vi "calibinformation.vi"(0 "object in":refnum<class "MBinteractive.lvclass">, 1 "校准点信息":u16[](array[numeric]), 5 "error in (no error)":errorcluster) -> (14 "object out":refnum<class "MBinteractive.lvclass">, 19 "error out":errorcluster)   [LabVIEW 2016, in "MBinteractive.lvclass"]
uses:
  MBinteractive.lvclass
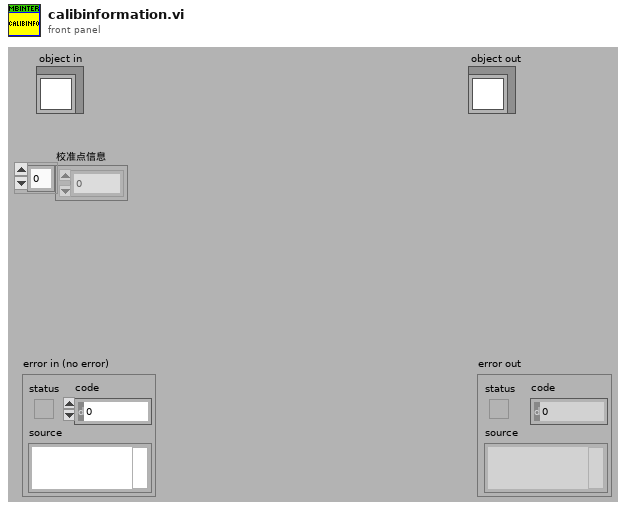
[diagram p1: front panel]
types:
  T1 = cluster{"低标液1浓度":dbl, "低标液1信号值":dbl, "低标液1启用":u16, "低标液2浓度":dbl, "低标液2信号值":dbl, "低标液2启用":u16, "低标液3浓度":dbl, "低标液3信号值":dbl, "低标液3启用":u16, "低标液4浓度":dbl, "低标液4信号值":dbl, "低标液4启用":u16, "低标液5浓度":dbl, "低标液5信号值":dbl, "低标液5启用":u16, "高标液1浓度":dbl, "高标液1信号值":dbl, "高标液1启用":u16, "高标液2浓度":dbl, "高标液2信号值":dbl, "高标液2启用":u16, "高标液3浓度":dbl, "高标液3信号值":dbl, "高标液3启用":u16, "高标液4浓度":dbl, "高标液4信号值":dbl, "高标液4启用":u16, "高标液5浓度":dbl, "高标液5信号值":dbl, "高标液5启用":u16, "低斜率":dbl, "低截距":dbl, "低二次多项式系数":dbl, "低线性相关系数":dbl, "高斜率":dbl, "高截距":dbl, "高二次多项式系数":dbl, "高线性相关系数":dbl}
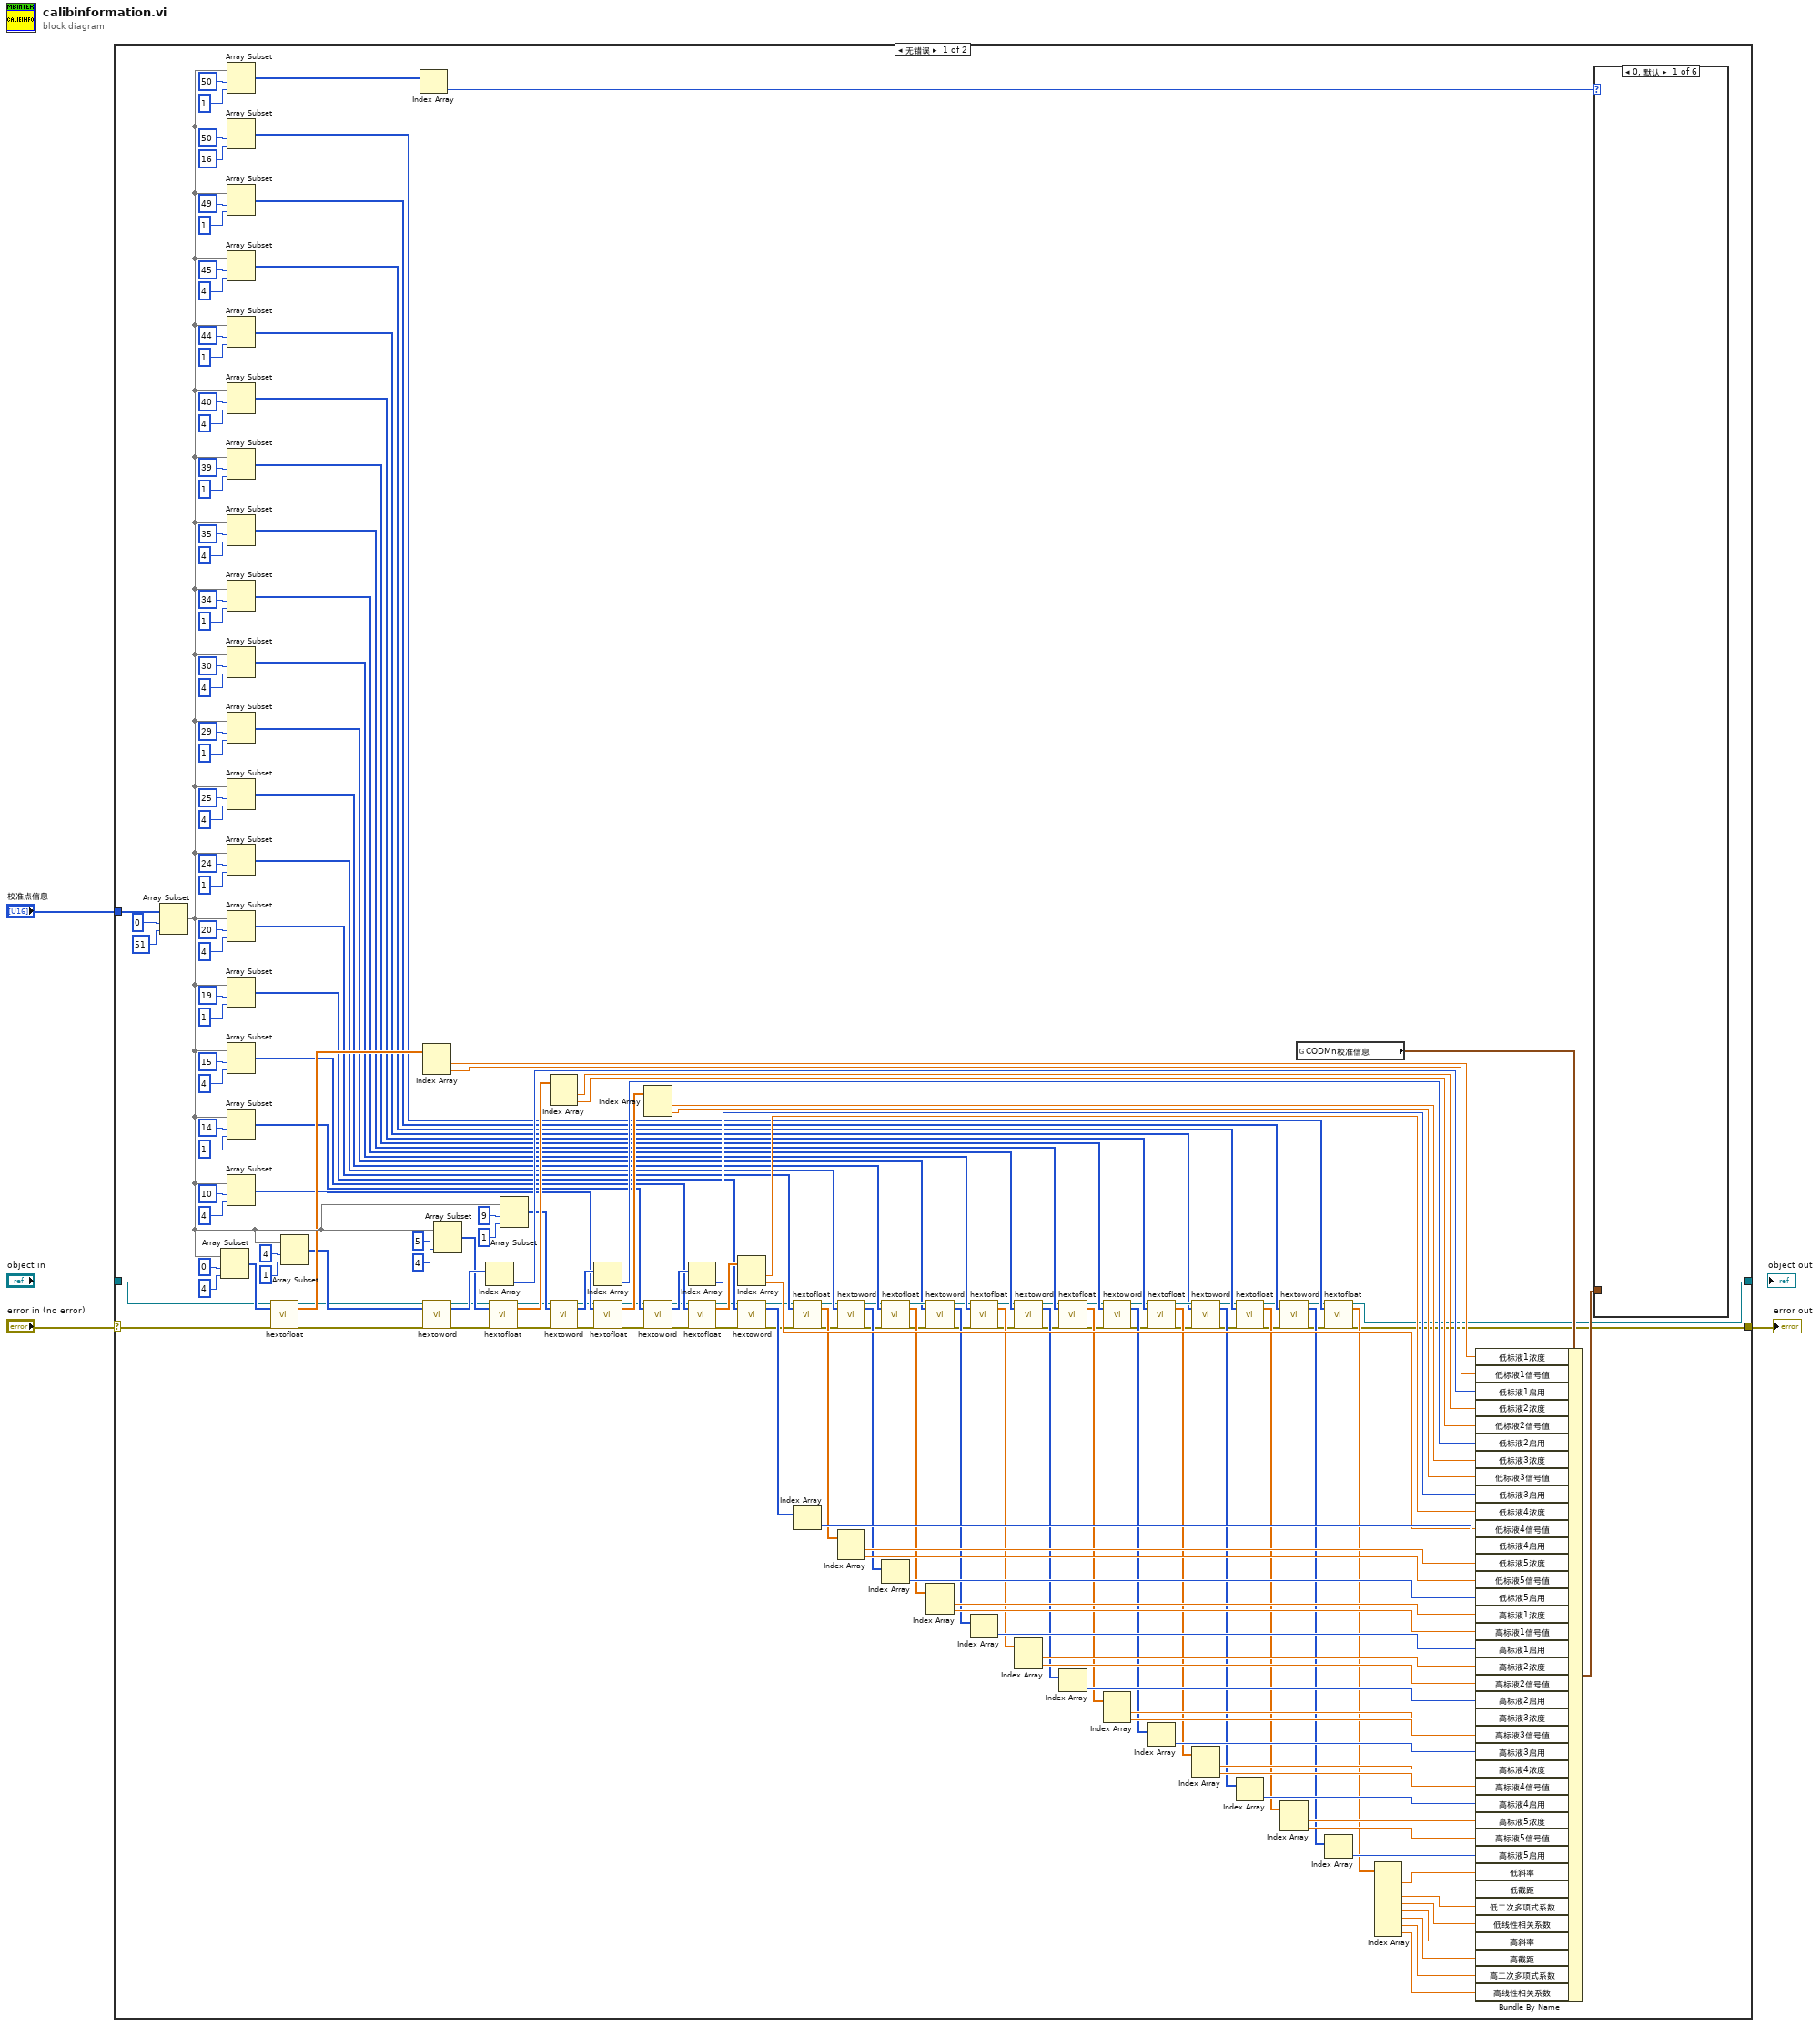
[diagram p0: block diagram]
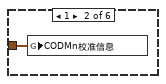
[diagram p2: hidden frame]
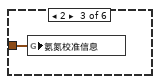
[diagram p3: hidden frame]
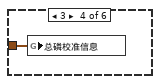
[diagram p4: hidden frame]
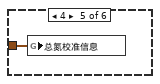
[diagram p5: hidden frame]
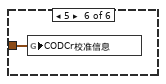
[diagram p6: hidden frame]
diagram:
  n1 = case shown="无错误" "error in (no error)" {
    selector: "error in (no error)" -> [w28 w188]
    tunnel: [w6 w188] -> w4
    tunnel: [w29 w187] -> w2
    tunnel: "object in" -> [w89 w187]
    tunnel: "校准点信息" -> [w93 _]
    frame No Error {
      n2 = Array Subset(array=w93, index=0 ("y"), length=51 ("长度")) -> (w173:u16[])
      n3 = Array Subset(array=w173, index=0 ("索引"), length=4 ("长度")) -> (w91:u16[])
      n4 = Array Subset(array=w173, index=50 ("索引"), length=1 ("长度")) -> (w170:u16[])
      n5 = Array Subset(array=w173, index=50 ("索引"), length=16 ("长度")) -> (w70:u16[])
      n6 = Array Subset(array=w173, index=49 ("索引"), length=1 ("长度")) -> (w58:u16[])
      n7 = Array Subset(array=w173, index=45 ("索引"), length=4 ("长度")) -> (w68:u16[])
      n8 = Array Subset(array=w173, index=44 ("索引"), length=1 ("长度")) -> (w34:u16[])
      n9 = Array Subset(array=w173, index=40 ("索引"), length=4 ("长度")) -> (w66:u16[])
      n10 = Array Subset(array=w173, index=39 ("索引"), length=1 ("长度")) -> (w38:u16[])
      n11 = Array Subset(array=w173, index=35 ("索引"), length=4 ("长度")) -> (w63:u16[])
      n12 = Array Subset(array=w173, index=34 ("索引"), length=1 ("长度")) -> (w42:u16[])
      n13 = Array Subset(array=w173, index=30 ("索引"), length=4 ("长度")) -> (w61:u16[])
      n14 = Array Subset(array=w173, index=29 ("索引"), length=1 ("长度")) -> (w45:u16[])
      n15 = Array Subset(array=w173, index=25 ("索引"), length=4 ("长度")) -> (w60:u16[])
      n16 = Array Subset(array=w173, index=24 ("索引"), length=1 ("长度")) -> (w56:u16[])
      n17 = Array Subset(array=w173, index=20 ("索引"), length=4 ("长度")) -> (w72:u16[])
      n18 = Array Subset(array=w173, index=19 ("索引"), length=1 ("长度")) -> (w74:u16[])
      n19 = Array Subset(array=w173, index=15 ("索引"), length=4 ("长度")) -> (w76:u16[])
      n20 = Array Subset(array=w173, index=14 ("索引"), length=1 ("长度")) -> (w78:u16[])
      n21 = Array Subset(array=w173, index=10 ("索引"), length=4 ("长度")) -> (w80:u16[])
      n22 = call-dynamic "hextofloat.vi"("object in"=w89, "数组"=w91, "error in (no error)"=w28) -> ("object out"=w87:refnum<class "MBinteractive.lvclass">, "FLOAT"=w90:sgl[], "error out"=w27:errorcluster)  [unwired: 14 in]
      n23 = Array Subset(array=w173, index=4 ("索引"), length=1 ("长度")) -> (w88:u16[])
      n24 = Index Array(array=w170) -> (element=w105:u16)  [unwired: 1 in]
      n25 = Index Array(array=w90) -> (element #1=w99:sgl, element #2=w100:sgl)  [unwired: 2 in]
      n26 = call-dynamic "hextoword.vi"("object in"=w87, "数组"=w88, "error in (no error)"=w27) -> ("object out"=w84:refnum<class "MBinteractive.lvclass">, "WORD"=w86:u16[], "error out"=w26:errorcluster)  [unwired: 14 in]
      n27 = Array Subset(array=w173, index=5 ("索引"), length=4 ("长度")) -> (w85:u16[])
      n28 = Index Array(array=w86) -> (element=w106:u16)  [unwired: 1 in]
      n29 = call-dynamic "hextofloat.vi"("object in"=w84, "数组"=w85, "error in (no error)"=w26) -> ("object out"=w54:refnum<class "MBinteractive.lvclass">, "FLOAT"=w83:sgl[], "error out"=w25:errorcluster)  [unwired: 14 in]
      n30 = Array Subset(array=w173, index=9 ("索引"), length=1 ("长度")) -> (w82:u16[])
      n31 = Index Array(array=w83) -> (element #1=w136:sgl, element #2=w137:sgl)  [unwired: 2 in]
      n32 = call-dynamic "hextoword.vi"("object in"=w54, "数组"=w82, "error in (no error)"=w25) -> ("object out"=w53:refnum<class "MBinteractive.lvclass">, "WORD"=w81:u16[], "error out"=w24:errorcluster)  [unwired: 14 in]
      n33 = Index Array(array=w81) -> (element=w138:u16)  [unwired: 1 in]
      n34 = call-dynamic "hextofloat.vi"("object in"=w53, "数组"=w80, "error in (no error)"=w24) -> ("object out"=w52:refnum<class "MBinteractive.lvclass">, "FLOAT"=w79:sgl[], "error out"=w23:errorcluster)  [unwired: 14 in]
      n35 = Index Array(array=w79) -> (element #1=w139:sgl, element #2=w140:sgl)  [unwired: 2 in]
      n36 = call-dynamic "hextoword.vi"("object in"=w52, "数组"=w78, "error in (no error)"=w23) -> ("object out"=w51:refnum<class "MBinteractive.lvclass">, "WORD"=w77:u16[], "error out"=w22:errorcluster)  [unwired: 14 in]
      n37 = Index Array(array=w77) -> (element=w141:u16)  [unwired: 1 in]
      n38 = call-dynamic "hextofloat.vi"("object in"=w51, "数组"=w76, "error in (no error)"=w22) -> ("object out"=w50:refnum<class "MBinteractive.lvclass">, "FLOAT"=w75:sgl[], "error out"=w21:errorcluster)  [unwired: 14 in]
      n39 = Index Array(array=w75) -> (element #1=w149:sgl, element #2=w150:sgl)  [unwired: 2 in]
      n40 = call-dynamic "hextoword.vi"("object in"=w50, "数组"=w74, "error in (no error)"=w21) -> ("object out"=w49:refnum<class "MBinteractive.lvclass">, "WORD"=w73:u16[], "error out"=w20:errorcluster)  [unwired: 14 in]
      n41 = call-dynamic "hextofloat.vi"("object in"=w49, "数组"=w72, "error in (no error)"=w20) -> ("object out"=w48:refnum<class "MBinteractive.lvclass">, "FLOAT"=w71:sgl[], "error out"=w18:errorcluster)  [unwired: 14 in]
      n42 = Index Array(array=w73) -> (element=w151:u16)  [unwired: 1 in]
      n43 = call-dynamic "hextoword.vi"("object in"=w48, "数组"=w56, "error in (no error)"=w18) -> ("object out"=w47:refnum<class "MBinteractive.lvclass">, "WORD"=w55:u16[], "error out"=w17:errorcluster)  [unwired: 14 in]
      n44 = Index Array(array=w71) -> (element #1=w152:sgl, element #2=w153:sgl)  [unwired: 2 in]
      n45 = call-dynamic "hextofloat.vi"("object in"=w47, "数组"=w60, "error in (no error)"=w17) -> ("object out"=w46:refnum<class "MBinteractive.lvclass">, "FLOAT"=w59:sgl[], "error out"=w16:errorcluster)  [unwired: 14 in]
      n46 = Index Array(array=w55) -> (element=w154:u16)  [unwired: 1 in]
      n47 = call-dynamic "hextoword.vi"("object in"=w46, "数组"=w45, "error in (no error)"=w16) -> ("object out"=w43:refnum<class "MBinteractive.lvclass">, "WORD"=w44:u16[], "error out"=w15:errorcluster)  [unwired: 14 in]
      n48 = Index Array(array=w59) -> (element #1=w155:sgl, element #2=w156:sgl)  [unwired: 2 in]
      n49 = call-dynamic "hextofloat.vi"("object in"=w43, "数组"=w61, "error in (no error)"=w15) -> ("object out"=w41:refnum<class "MBinteractive.lvclass">, "FLOAT"=w62:sgl[], "error out"=w14:errorcluster)  [unwired: 14 in]
      n50 = Index Array(array=w44) -> (element=w157:u16)  [unwired: 1 in]
      n51 = call-dynamic "hextoword.vi"("object in"=w41, "数组"=w42, "error in (no error)"=w14) -> ("object out"=w39:refnum<class "MBinteractive.lvclass">, "WORD"=w40:u16[], "error out"=w13:errorcluster)  [unwired: 14 in]
      n52 = Index Array(array=w62) -> (element #1=w158:sgl, element #2=w159:sgl)  [unwired: 2 in]
      n53 = call-dynamic "hextofloat.vi"("object in"=w39, "数组"=w63, "error in (no error)"=w13) -> ("object out"=w36:refnum<class "MBinteractive.lvclass">, "FLOAT"=w64:sgl[], "error out"=w12:errorcluster)  [unwired: 14 in]
      n54 = Index Array(array=w40) -> (element=w160:u16)  [unwired: 1 in]
      n55 = call-dynamic "hextoword.vi"("object in"=w36, "数组"=w38, "error in (no error)"=w12) -> ("object out"=w19:refnum<class "MBinteractive.lvclass">, "WORD"=w37:u16[], "error out"=w11:errorcluster)  [unwired: 14 in]
      n56 = Index Array(array=w64) -> (element #1=w161:sgl, element #2=w162:sgl)  [unwired: 2 in]
      n57 = call-dynamic "hextofloat.vi"("object in"=w19, "数组"=w66, "error in (no error)"=w11) -> ("object out"=w35:refnum<class "MBinteractive.lvclass">, "FLOAT"=w65:sgl[], "error out"=w10:errorcluster)  [unwired: 14 in]
      n58 = Index Array(array=w37) -> (element=w163:u16)  [unwired: 1 in]
      n59 = call-dynamic "hextoword.vi"("object in"=w35, "数组"=w34, "error in (no error)"=w10) -> ("object out"=w32:refnum<class "MBinteractive.lvclass">, "WORD"=w33:u16[], "error out"=w9:errorcluster)  [unwired: 14 in]
      n60 = Index Array(array=w65) -> (element #1=w164:sgl, element #2=w165:sgl)  [unwired: 2 in]
      n61 = call-dynamic "hextofloat.vi"("object in"=w32, "数组"=w68, "error in (no error)"=w9) -> ("object out"=w31:refnum<class "MBinteractive.lvclass">, "FLOAT"=w67:sgl[], "error out"=w8:errorcluster)  [unwired: 14 in]
      n62 = Index Array(array=w33) -> (element=w166:u16)  [unwired: 1 in]
      n63 = call-dynamic "hextoword.vi"("object in"=w31, "数组"=w58, "error in (no error)"=w8) -> ("object out"=w30:refnum<class "MBinteractive.lvclass">, "WORD"=w57:u16[], "error out"=w7:errorcluster)  [unwired: 14 in]
      n64 = Index Array(array=w67) -> (element #1=w167:sgl, element #2=w168:sgl)  [unwired: 2 in]
      n65 = global read "全局1.vi" "CODMn校准信息"() -> (w92:T1)
      n66 = call-dynamic "hextofloat.vi"("object in"=w30, "数组"=w70, "error in (no error)"=w7) -> ("object out"=w29:refnum<class "MBinteractive.lvclass">, "FLOAT"=w69:sgl[], "error out"=w6:errorcluster)  [unwired: 14 in]
      n67 = Index Array(array=w57) -> (element=w169:u16)  [unwired: 1 in]
      n68 = Index Array(array=w69) -> (element #1=w174:sgl, element #2=w175:sgl, element #3=w176:sgl, element #4=w177:sgl, element #5=w178:sgl, element #6=w179:sgl, element #7=w180:sgl, element #8=w181:sgl)  [unwired: 8 in]
      n69 = Bundle By Name(cluster=w92, "低标液1浓度"=w99, "低标液1信号值"=w100, "低标液1启用"=w106, "低标液2浓度"=w136, "低标液2信号值"=w137, "低标液2启用"=w138, "低标液3浓度"=w139, "低标液3信号值"=w140, "低标液3启用"=w141, "低标液4浓度"=w149, "低标液4信号值"=w150, "低标液4启用"=w151, "低标液5浓度"=w152, "低标液5信号值"=w153, "低标液5启用"=w154, "高标液1浓度"=w155, "高标液1信号值"=w156, "高标液1启用"=w157, "高标液2浓度"=w158, "高标液2信号值"=w159, "高标液2启用"=w160, "高标液3浓度"=w161, "高标液3信号值"=w162, "高标液3启用"=w163, "高标液4浓度"=w164, "高标液4信号值"=w165, "高标液4启用"=w166, "高标液5浓度"=w167, "高标液5信号值"=w168, "高标液5启用"=w169, "低斜率"=w174, "低截距"=w175, "低二次多项式系数"=w176, "低线性相关系数"=w177, "高斜率"=w178, "高截距"=w179, "高二次多项式系数"=w180, "高线性相关系数"=w181) -> (w94:T1)
      n70 = case shown="0, 默认" w105 {
        tunnel: w94 -> [_ w182 w183 w184 w185 w186]
        frame 0, Default {
        }
        frame 1 {
          n71 = global write "全局1.vi" "CODMn校准信息"(w182) -> ()
        }
        frame 2 {
          n72 = global write "全局1.vi" "氨氮校准信息"(w183) -> ()
        }
        frame 3 {
          n73 = global write "全局1.vi" "总磷校准信息"(w184) -> ()
        }
        frame 4 {
          n74 = global write "全局1.vi" "总氮校准信息"(w185) -> ()
        }
        frame 5 {
          n75 = global write "全局1.vi" "CODCr校准信息"(w186) -> ()
        }
      }
    }
    frame Error {
    }
  }
  "error out" <- w4
  "object out" <- w2
